vi "Log in and Post.vi"() -> ()   [LabVIEW 2022 SP3]
uses:
  firebase.lvclass
panel:
  in  "Data":T1 {"Dial" scale=0.0..10.0}
  in  "endPoint":string
  out "firebase out":refnum<class "firebase.lvclass">
  in  "Email":string
  in  "Password":string
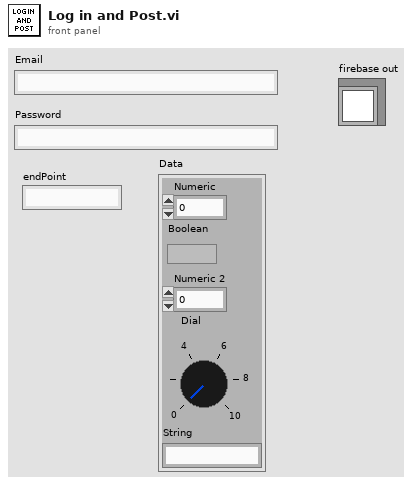
[diagram p1: front panel]
types:
  T1 = cluster{"Numeric":dbl, "Boolean":bool, "Numeric 2":dbl, "Dial":dbl, "String":string}
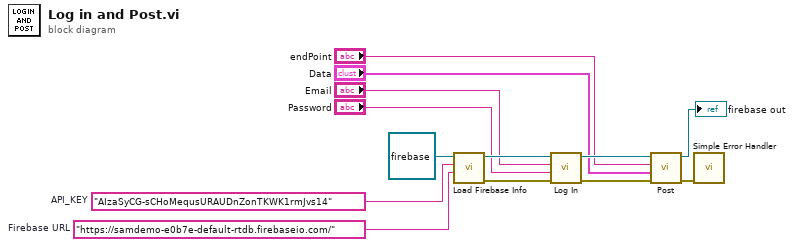
[diagram p0: block diagram]
diagram:
  w1 = "AIzaSyCG-sCHoMequsURAUDnZonTKWK1rmJvs14"  # API_KEY
  w2 = "https://samdemo-e0b7e-default-rtdb.firebaseio.com/"  # Firebase URL
  n1 = call "Load Firebase Info.vi"("Firebase URL"=w2, "API_KEY"=w1, "firebase in"=refnum<class "firebase.lvclass"> refnum ("firebase.lvclass")) -> ("error out"=w13:errorcluster, "firebase out"=w9:refnum<class "firebase.lvclass">)  [unwired: 7 in]
  n2 = call-dynamic "Log In.vi"("error in"=w13, "password"="Password", "email"="Email", "firebase in"=w9) -> ("error out"=w12:errorcluster, "firebase out"=w6:refnum<class "firebase.lvclass">)  [unwired: 6 in]
  n3 = call-dynamic "Post.vi"("error in"=w12, "Anything"="Data", "endPoint"="endPoint", "firebase in"=w6) -> ("error out"=w11:errorcluster, "firebase out"=→"firebase out":refnum<class "firebase.lvclass">)  [unwired: 5 in, 1 out]
  n4 = call <vilib>:"Simple Error Handler.vi"("error in (no error)"=w11) -> ()  [unwired: 4 in, 5 out]
